vi "RenderPoint.vi"(8 "No Error":errorcluster, 9 "y":sgl, 10 "x":sgl, 11 "renderer [SDL_Renderer *]":i64) -> (0 "error out":errorcluster)   [LabVIEW 2024, in "SDL3.lvlib" / "Render.lvlib"]
doc: "Draw a point on the current rendering target at subpixel precision."
uses:
  Render.lvlib
  Error/Error.lvlib
  _LV-SDL3/Lib/SDL3-32.dll
panel:
  # "https://wiki.libsdl.org/SDL3/SDL_RenderPoint"
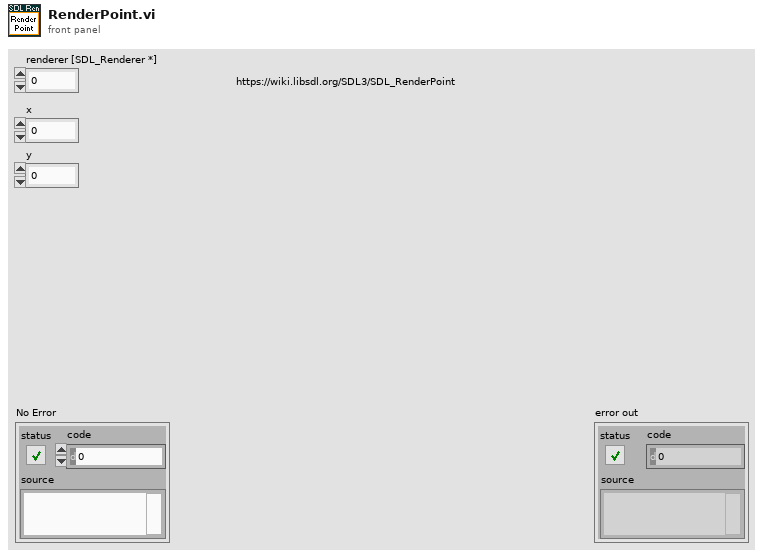
[diagram p1: front panel]
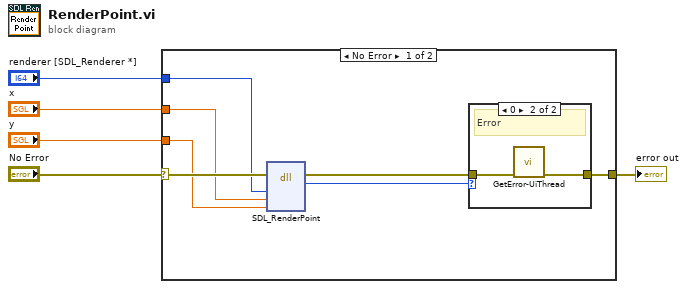
[diagram p0: block diagram]
diagram:
  n1 = case shown="No Error" "No Error" {
    selector: "No Error" -> [w12 w16]
    tunnel: [w10 w16] -> w4
    tunnel: "renderer [SDL_Renderer *]" -> [w8 _]
    tunnel: "x" -> [w7 _]
    tunnel: "y" -> [w6 _]
    frame No Error {
      n2 = dll-call lib="C:/Users/Thomas/Documents/Projects/_LV-SDL3/Lib/SDL3-*.*" fn="SDL_RenderPoint"(error in=w12, "renderer"=w8, "x"=w7, "y"=w6) -> (error out=w11:errorcluster, "return type"=w9:i32)  [unwired: 5 in, 1 out]
      n3 = case shown="0" w9 {
        tunnel: w11 -> [w13 w15]
        tunnel: [w13 w14] -> w10
        frame Default {
          # "Ok"
        }
        frame 0 {
          # "Error"
          n4 = call "GetError-UiThread.vi"("No Error"=w15) -> ("error out"=w14:errorcluster)  [unwired: 10 in]
        }
      }
    }
    frame Error {
    }
  }
  "error out" <- w4
